vi "Data Parsing.vi"(8 "error in":errorcluster, 10 "Data Read":string, 11 "TCP in":refnum<class "TCP.lvclass">) -> (0 "error out":errorcluster, 1 "Graph Data":T1, 2 "Data Out":string[](array[string]), 3 "TCP out":refnum<class "TCP.lvclass">)   [LabVIEW 2021, in "TCP.lvclass"]
uses:
  TCP.lvclass
  controls/Data for Graph.ctl
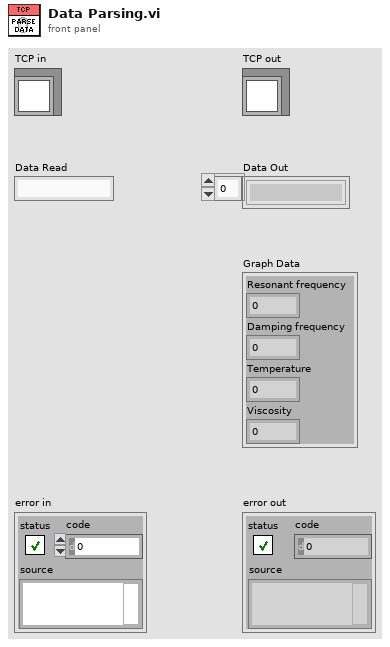
[diagram p1: front panel]
types:
  T1 = typedef "Data for Graph.ctl" = cluster{"Resonant frequency":dbl, "Damping frequency":dbl, "Temperature":dbl, "Viscosity":dbl}
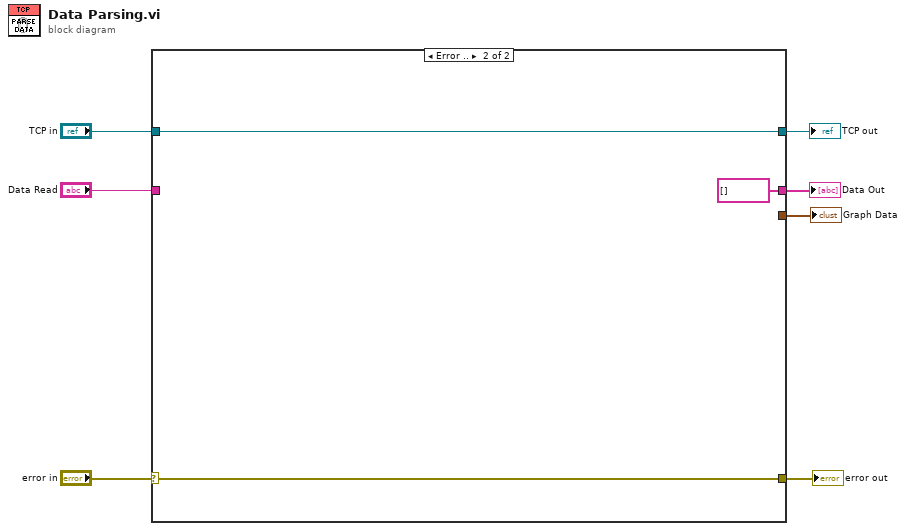
[diagram p0: block diagram]
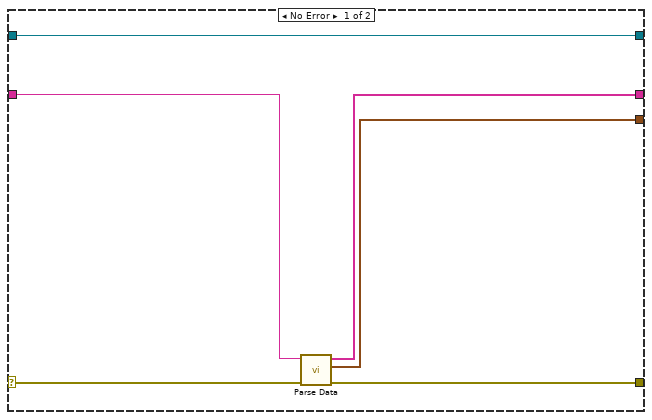
[diagram p2: hidden frame]
diagram:
  n1 = case shown="Error .." "error in" {
    selector: "error in" -> [w12 w15]
    tunnel: "TCP in" -> [w13 w16]
    tunnel: [w13 w16] -> w5
    tunnel: "Data Read" -> [w11 _]
    tunnel: [w10 w15] -> w3
    tunnel: [w9 string[] [] ("Data Out")] -> w2
    tunnel: [w8 _] -> w1
    frame No Error {
      n2 = call "Parse Data.vi"("error in"=w12, "Data Read"=w11) -> ("error out"=w10:errorcluster, "Graph Data out"=w8:T1, "Data Out"=w9:string[])  [unwired: 7 in]
    }
    frame Error {
    }
  }
  "error out" <- w3
  "TCP out" <- w5
  "Data Out" <- w2
  "Graph Data" <- w1
